vi "Array of U32_Read Index.vi"(9 "Default":u32[](array[numeric]), 11 "Index":i32) -> (1 "Value":u32[](array[numeric]))   [LabVIEW 2020, in "Current Value Table(Rebuild).lvlib"]
doc: "This VI takes a memory index (I32) and will perform a read on that index. This VI will never return the default value, as it has no error handling for increased performance. If the index is invalid, the default for the data type will be returned."
uses:
  Current Value Table(Rebuild).lvlib
  Type Defs/Memory Commands.ctl
  Array of U32_Memory Block.vi
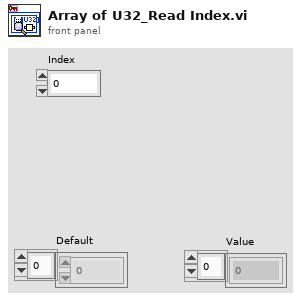
[diagram p1: front panel]
types:
  T1 = typedef "Current Value Table(Rebuild).lvlib/Memory Commands.ctl" = enum16{"Init", "Add Data", "Read", "Read Group", "Read All", "Write", "Write Group", "Get Size"}
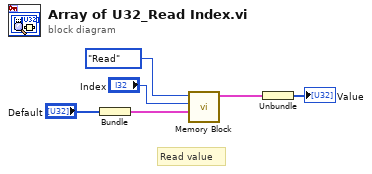
[diagram p0: block diagram]
diagram:
  # "Read value"
  n1 = Bundle("Default"="Default") -> (w4:cluster{"Default":u32[]})  [unwired: 1 in]
  n2 = call-poly "Memory Block.vi"("Value"=w4, "Index"="Index", "Method"=Memory_Commands."Read") -> ("Value Out"=w2:cluster{"U32 Array":u32[]})  [unwired: 6 in, 2 out]
  n3 = Unbundle(w2) -> ("U32 Array"=→"Value":u32[])
